vi "复制.vi"() -> ()   [LabVIEW 2018]
panel:
  out "新路径":path
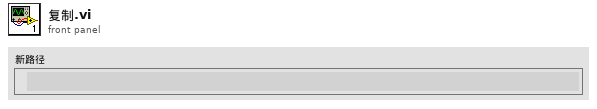
[diagram p1: front panel]
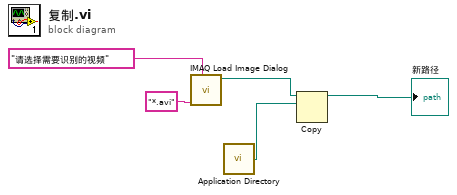
[diagram p0: block diagram]
diagram:
  n1 = call "IMAQ Load Image Dialog"("Prompt"="请选择需要识别的视频" ("prompt"), "Pattern"="*.avi") -> ("Path"=w3:path)  [unwired: 7 in, 2 out]
  n2 = call <vilib>:"Application Directory.vi"() -> ("Application Directory"=w2:path)
  n3 = Copy(10:w2, 11:w3) -> (3:→"新路径":path)  [unwired: 3 in, 2 out]
